vi "Teardown.vi"(8 "Error In":errorcluster, 11 "VI In":refnum<vi>) -> (0 "Error Out":errorcluster, 3 "VI Out":refnum<vi>)   [LabVIEW 2017, in "Toolkit.lvlib" / "Tests.lvlib"]
uses:
  Tests.lvlib
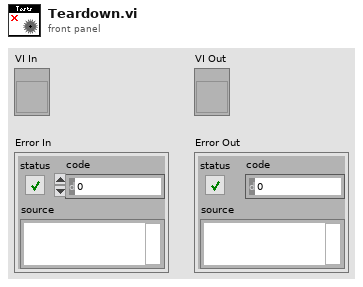
[diagram p1: front panel]
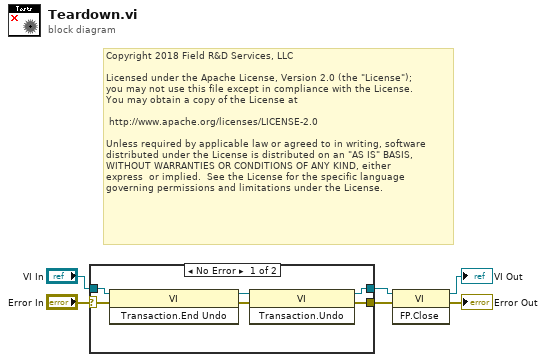
[diagram p0: block diagram]
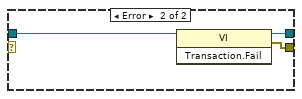
[diagram p2: hidden frame]
diagram:
  # "Copyright 2018 Field R&D Services, LLC\n\nLicensed under the Apache License, Version 2.0 (the \"License\");\nyou may not use this file except in compliance with the License.\nYou may obtain a copy of the License at\n\n\thttp://www.apache.org/licenses/LICENSE-2.0\n\nUnless required by applicable law or agreed to in writing, software\ndistributed under the License is distributed on an \"AS IS\" BASIS,\nWITHOUT WARRANTIES OR CONDITIONS OF ANY KIND, either \nexpress  or implied.  See the License for the specific language \ngoverning permissions and limitations under the License."
  n1 = case shown="No Error" "Error In" {
    selector: "Error In" -> [w10 _]
    tunnel: [w12 w13] -> w4
    tunnel: [w11 w14] -> w3
    tunnel: "VI In" -> [w9 w15]
    frame No Error {
      n2 = invoke class="VI" method="Transaction.End Undo"(reference=w9, error in=w10) -> (reference out=w8:refnum<vi>, error out=w7:errorcluster)  [unwired: 1 in, 1 out]
      n3 = invoke class="VI" method="Transaction.Undo"(reference=w8, error in=w7) -> (reference out=w11:refnum<vi>, error out=w12:errorcluster)  [unwired: 1 in, 1 out]
    }
    frame Error {
      n4 = invoke class="VI" method="Transaction.Fail"(reference=w15) -> (reference out=w14:refnum<vi>, error out=w13:errorcluster)  [unwired: 2 in, 1 out]
    }
  }
  n5 = invoke class="VI" method="FP.Close"(reference=w3, error in=w4) -> (reference out=→"VI Out":refnum<vi>, error out=→"Error Out":errorcluster)  [unwired: 1 in, 1 out]
